vi "Giffler Thompson Active Schedule Engine.vi"(8 "Number of  Jobs":i32=4, 9 "Number of Machines":i32=4, 10 "Processing Times":u16[][](array[numeric])=[[34, 15, 38, 95], [2, 89, 19, 7], [54, 70, 28, 34], [61, 9, 87, 29]], 11 "Schedule In":u16[](array[numeric])=[12, 0, 7, 2, 6, 3, 13, 5, 1, 4, 14, 11, 10, 15, 8, 9]) -> (0 "Machine Completion Times":u16[](array[numeric]), 1 "Job Completion Times":u16[](array[numeric]), 2 "Completion Times":u16[][](array[numeric]), 3 "Start Times":u16[][](array[numeric]), 4 "Ordered Schedule Out":u16[](array[numeric]))   [LabVIEW 2013, in "Scheduler.lvclass"]
uses:
  Scheduler.lvclass
  Prins FIFO Scheduler Methods and Controls/Controls/Prins FIFO Scheduler Result Cluster.ctl
panel:
  out "error out":errorcluster
  out "Graph Out":picture
  in  "error in (no error)":errorcluster
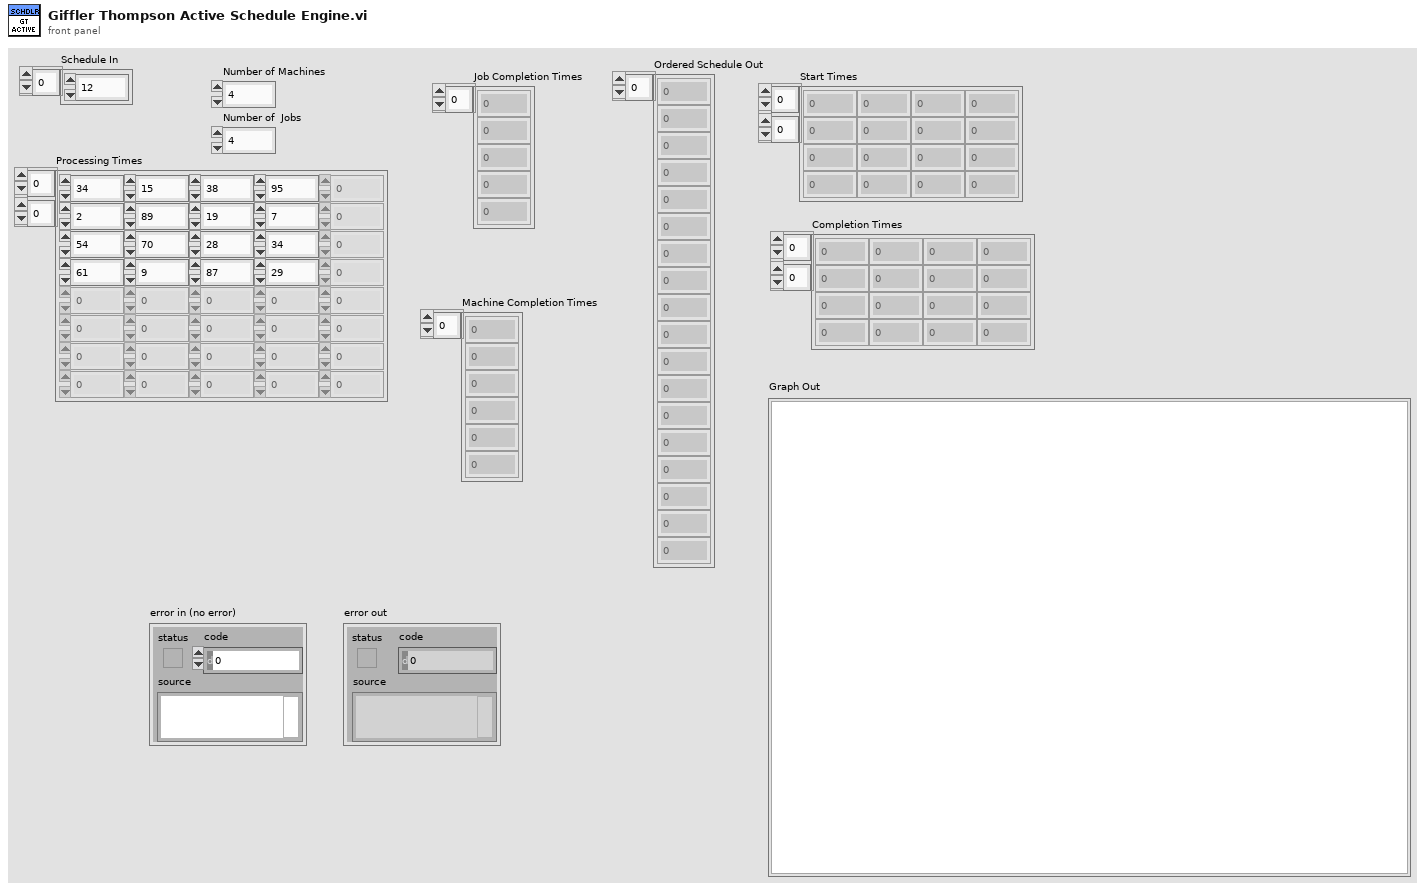
[diagram p1: front panel]
types:
  T1 = typedef "Scheduler.lvclass/Prins FIFO Scheduler Result Cluster.ctl" = cluster{"Start Times":u16[][], "Completion Times":u16[][], "Processing Times":u16[][]}
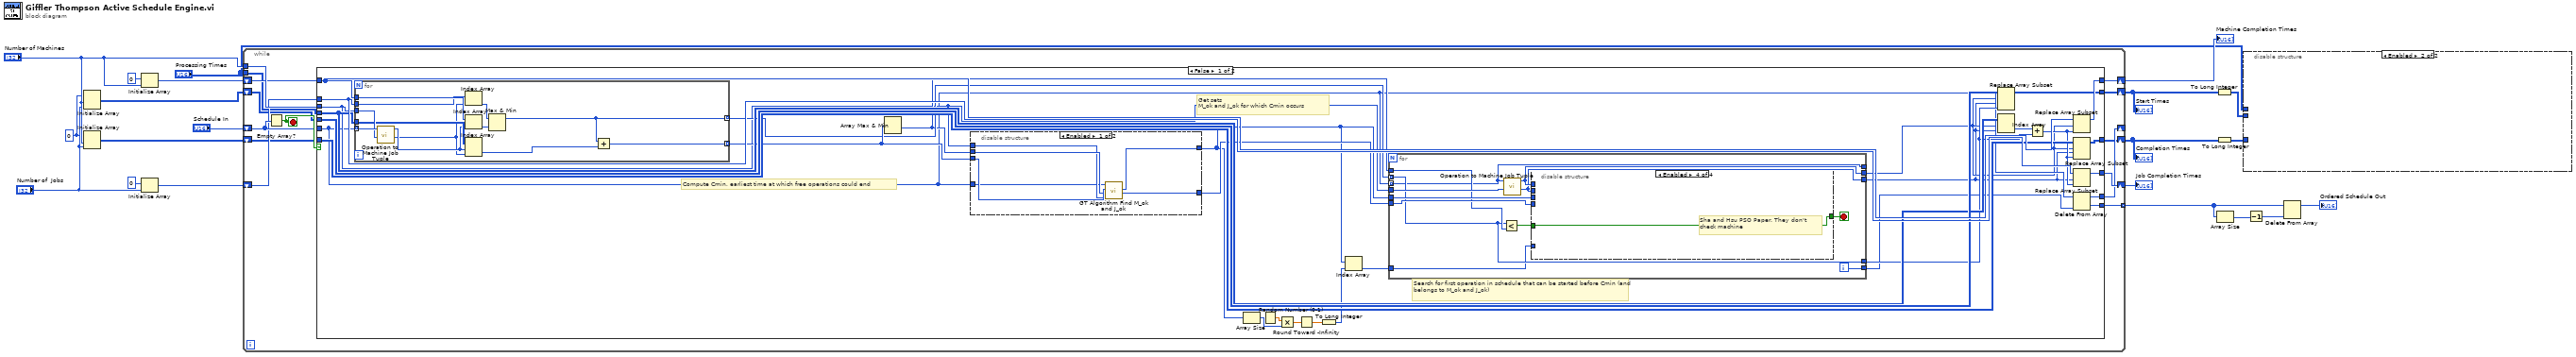
[diagram p0: block diagram]
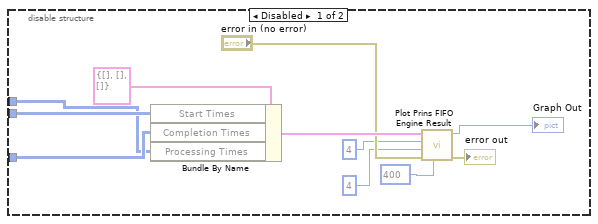
[diagram p2: hidden frame]
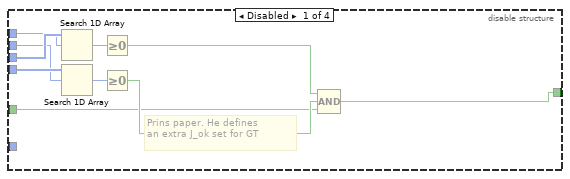
[diagram p4: hidden frame]
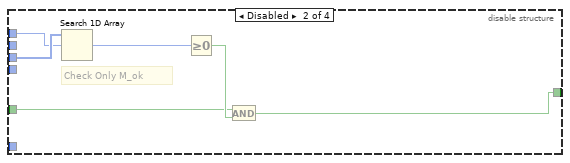
[diagram p5: hidden frame]
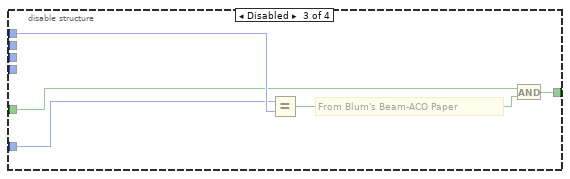
[diagram p6: hidden frame]
diagram:
  w12 = u16 0 ("element")
  n1 = Initialize Array(w12, "Number of Machines", "Number of  Jobs") -> (w11:u16[][])
  n2 = Initialize Array(w12, "Number of Machines", "Number of  Jobs") -> (w2:u16[][])
  n3 = Initialize Array(u16 0 ("element"), "Number of Machines") -> (w18:u16[])
  n4 = Initialize Array(u16 0 ("element"), "Number of  Jobs") -> (w19:u16[])
  n5 = while {
    shift-right: [w27] -> _
    shift-left: "Schedule In" -> [w34]
    tunnel: "Number of Machines" -> [w33]
    shift-right: [w30] -> w17
    shift-left: w19 -> [w32]
    shift-right: [w29] -> w16
    shift-left: w18 -> [w31]
    shift-right: [w25] -> w4
    shift-left: w2 -> [w26]
    tunnel: "Processing Times" -> [w28]
    shift-right: [w23] -> w6
    shift-left: w11 -> [w24]
    tunnel: [w22] -> w7 mode=indexing
    stop <- w35 stop-if-true
    n6 = Empty Array?(array=w34) -> (empty?=w35:bool)
    n7 = case shown="False" w35 {
      tunnel: w34 -> [w46 w120]
      tunnel: w33 -> [w48 _]
      tunnel: w32 -> [w64 w122]
      tunnel: w31 -> [w65 w121]
      tunnel: [w63 w122] -> w30
      tunnel: [w62 w121] -> w29
      tunnel: w28 -> [w57 _]
      tunnel: [w51 w120] -> w27
      tunnel: w26 -> [w61 w119]
      tunnel: [w60 w119] -> w25
      tunnel: w24 -> [w59 w118]
      tunnel: [w58 w118] -> w23
      tunnel: [w50 _] -> w22
      frame False {
        # "Search for first operation in schedule that can be started before Cmin (and belongs to M_ok and J_ok)"
        # "Get sets \nM_ok and J_ok for which Cmin occurs"
        # "Compute Cmin, earliest time at which free operations could end"
        n8 = for {
          tunnel: w46 -> [w117] mode=indexing
          tunnel: w48 -> [w116]
          tunnel: w64 -> [w114]
          tunnel: w65 -> [w115]
          tunnel: [w107] -> w55 mode=indexing
          tunnel: w57 -> [w111]
          tunnel: [w106] -> w54 mode=indexing
          n9 = call "Operation to Machine Job Tuple.vi"("Number of Machines"=w116, "Operation Number"=w117) -> ("Job No"=w109:i32, "Machine No"=w110:i32)  [unwired: 8 in]
          n10 = Index Array(array=w114, index=w109) -> (element=w113:u16)
          n11 = Index Array(array=w115, index=w110) -> (element=w112:u16)
          n12 = Index Array(array=w111, index (row)=w110, index (col)=w109) -> (element=w108:u16)
          n13 = Max & Min(x=w113, y=w112) -> (max(x,y)=w106:u16)  [unwired: 1 out]
          n14 = Add(x=w106, y=w108) -> (x+y=w107:u16)
        }
        n15 = Array Max & Min(array=w55) -> (min value=w49:u16)  [unwired: 3 out]
        n16 = disable-structure shown="Enabled" {
          disable-tunnel: w55 -> [w71 _]
          disable-tunnel: w49 -> [w70 _]
          disable-tunnel: w48 -> [w69 _]
          disable-tunnel: [w68 _] -> w47
          disable-tunnel: [w67 _] -> w37
          disable-tunnel: w46 -> [w66 _]
          frame Enabled {
            n17 = call "GT Algorithm Find M_ok and J_ok.vi"("Number of Machines"=w69, "Cmin"=w70, "Cmin Array"=w71, "Schedule In"=w66) -> ("J_ok(Jobs)"=w68:i32[], "M_ok(Machines)"=w67:i32[])  [unwired: 6 in]
          }
          frame Disabled {
          }
        }
        n18 = Array Size(array=w37) -> (size(s)=w41:i32)
        n19 = Random Number (0-1)() -> (number: 0 to 1=w42:dbl)
        n20 = Multiply(x=w42, y=w41) -> (x*y=w40:dbl)
        n21 = Round Toward -Infinity(1:w40) -> (0:w39:dbl)
        n22 = To Long Integer(number=w39) -> (32bit integer=w38:i32)
        n23 = Index Array(array=w37, index=w38) -> (element=w36:i32)
        n24 = for {
          tunnel: w46 -> [w76] mode=indexing
          tunnel: w48 -> [w83]
          tunnel: w54 -> [w77] mode=indexing
          tunnel: w37 -> [w82]
          tunnel: w47 -> [w81]
          tunnel: w49 -> [w80]
          tunnel: [w77] -> w56
          tunnel: [w76] -> _
          tunnel: [w75] -> w45
          tunnel: [w74] -> w44
          tunnel: [w73] -> w43
          tunnel: w36 -> [w72]
          i -> [w73]
          stop <- w78 stop-if-true
          n25 = Less?(x=w77, y=w80) -> (x < y?=w79:bool)
          n26 = call "Operation to Machine Job Tuple.vi"("Number of Machines"=w83, "Operation Number"=w76) -> ("Job No"=w74:i32, "Machine No"=w75:i32)  [unwired: 8 in]
          n27 = disable-structure shown="Enabled" {
            disable-tunnel: w82 -> [w93 w99 _ _]
            disable-tunnel: w81 -> [w91 _ _ _]
            disable-tunnel: w79 -> [w87 w95 w101 w105]
            disable-tunnel: [w86 w94 w100 w105] -> w78
            disable-tunnel: w75 -> [w85 w98 w104 _]
            disable-tunnel: w74 -> [w84 _ _ _]
            disable-tunnel: w72 -> [_ _ w103 _]
            frame Disabled {
              # "Prins paper. He defines\nan extra J_ok set for GT"
              n28 = Search 1D Array(1D array=w93, element=w85) -> (index of element=w92:i32)  [unwired: 1 in]
              n29 = Search 1D Array(1D array=w91, element=w84) -> (index of element=w90:i32)  [unwired: 1 in]
              n30 = Greater Or Equal To 0?(x=w92) -> (x >= 0?=w89:bool)
              n31 = Greater Or Equal To 0?(x=w90) -> (x >= 0?=w88:bool)
              n32 = Compound Arithmetic op=AND(w89, w88, w87) -> (w86:bool)
            }
            frame Disabled {
              # "Check Only M_ok"
              n33 = Search 1D Array(1D array=w99, element=w98) -> (index of element=w97:i32)  [unwired: 1 in]
              n34 = Greater Or Equal To 0?(x=w97) -> (x >= 0?=w96:bool)
              n35 = And(x=w95, y=w96) -> (x .and. y?=w94:bool)
            }
            frame Disabled {
              # "From Blum's Beam-ACO Paper"
              n36 = Equal?(x=w103, y=w104) -> (x = y?=w102:bool)
              n37 = And(x=w101, y=w102) -> (x .and. y?=w100:bool)
            }
            frame Enabled {
              # "Sha and Hsu PSO Paper. They don't\ncheck machine"
            }
          }
        }
        n38 = Replace Array Subset(array=w59, new element=w56, index (row)=w45, index (col)=w44) -> (w58:u16[][])
        n39 = Index Array(array=w57, index (row)=w45, index (col)=w44) -> (element=w53:u16)
        n40 = Add(x=w53, y=w56) -> (x+y=w52:u16)
        n41 = Replace Array Subset(array=w65, new element=w52, index=w45) -> (w62:u16[])
        n42 = Replace Array Subset(array=w61, new element=w52, index (row)=w45, index (col)=w44) -> (w60:u16[][])
        n43 = Replace Array Subset(array=w64, new element=w52, index=w44) -> (w63:u16[])
        n44 = Delete From Array(array=w46, index=w43) -> (deleted portion=w50:u16, array with subset deleted=w51:u16[])  [unwired: 1 in]
      }
      frame True {
      }
    }
  }
  "Completion Times" <- w4
  "Job Completion Times" <- w17
  "Machine Completion Times" <- w16
  "Start Times" <- w6
  n45 = To Long Integer(number=w6) -> (32bit integer=w5:i32[][])
  n46 = To Long Integer(number=w4) -> (32bit integer=w3:i32[][])
  n47 = Array Size(array=w7) -> (size(s)=w10:i32)
  n48 = disable-structure shown="Enabled" {
    disable-tunnel: w5 -> [w126 _]
    disable-tunnel: w3 -> [w125 _]
    disable-tunnel: "Processing Times" -> [w123 _]
    frame Disabled {
      n49 = Bundle By Name(cluster=T1 {"Start Times"=[], "Completion Times"=[], "Processing Times"=[]} ("FIFO Results"), "Start Times"=w126, "Completion Times"=w125, "Processing Times"=w123) -> (w132:T1)
      n50 = call "Plot Prins FIFO Engine Result.vi"("Plot Max Value"=400, "error in (no error)"="error in (no error)", "Number of Jobs"=4, "Number of Machines"=4, "FIFO Results"=w132) -> ("error out"=→"error out":errorcluster, "Graph Out"=→"Graph Out":picture)  [unwired: 5 in]
    }
    frame Enabled {
    }
  }
  n51 = Decrement(x=w10) -> (x-1=w9:i32)
  n52 = Delete From Array(array=w7, index=w9) -> (array with subset deleted=→"Ordered Schedule Out":u16[])  [unwired: 1 in, 1 out]
